vi "DEMPViewer.vi"() -> ()   [LabVIEW 2024]
uses:
  <vilib>/Utility/file.llb/Write Delimited Spreadsheet (string).vi
  E:/CodeProjects/DEMPViewer/ClassLibrary1.dll
  ClassLibrary1.dll
panel:
  out "SelectedAnalytes":string[](array[string])
  in  "Analytes":i32[](listbox)
  in  "Maximum":dbl=70.0
  in  "X Limits":bool
  in  "Minimum":dbl
  in  "Copy":bool
  out "Table Control":string[][](table)
  out "Y Scale":i64
  out "Selected Bias":i64
  in  "Clip Ends":bool=TRUE
  in  "10 nA":bool
  in  "5nA":bool
  in  "3nA":bool
  in  "1nA":bool
  in  "Y Limits":bool
  in  "500 mV":bool
  in  "100 mV":bool
  in  "50 mV":bool
  in  "10 mV":bool
  in  "Bias":bool
  in  "SaveDown":bool
  in  "LoadDown":bool
  out "Currently Loading":string
  in  "Refresh":bool
  out "Bias Graph":cluster{dbl[], "Data":dbl[]}[](graph)
  out "XY Graph 32":cluster{dbl[], "Data":dbl[]}[](graph)
  out "XY Graph 31":cluster{dbl[], "Data":dbl[]}[](graph)
  out "XY Graph 30":cluster{dbl[], "Data":dbl[]}[](graph)
  out "XY Graph 29":cluster{dbl[], "Data":dbl[]}[](graph)
  out "XY Graph 28":cluster{dbl[], "Data":dbl[]}[](graph)
  out "XY Graph 27":cluster{dbl[], "Data":dbl[]}[](graph)
  out "XY Graph 26":cluster{dbl[], "Data":dbl[]}[](graph)
  out "XY Graph 25":cluster{dbl[], "Data":dbl[]}[](graph)
  out "XY Graph 24":cluster{dbl[], "Data":dbl[]}[](graph)
  out "XY Graph 23":cluster{dbl[], "Data":dbl[]}[](graph)
  out "XY Graph 22":cluster{dbl[], "Data":dbl[]}[](graph)
  out "XY Graph 21":cluster{dbl[], "Data":dbl[]}[](graph)
  out "XY Graph 20":cluster{dbl[], "Data":dbl[]}[](graph)
  out "XY Graph 19":cluster{dbl[], "Data":dbl[]}[](graph)
  out "XY Graph 18":cluster{dbl[], "Data":dbl[]}[](graph)
  out "XY Graph 17":cluster{dbl[], "Data":dbl[]}[](graph)
  out "XY Graph 16":cluster{dbl[], "Data":dbl[]}[](graph)
  out "XY Graph 15":cluster{dbl[], "Data":dbl[]}[](graph)
  out "XY Graph 14":cluster{dbl[], "Data":dbl[]}[](graph)
  out "XY Graph 13":cluster{dbl[], "Data":dbl[]}[](graph)
  out "XY Graph 12":cluster{dbl[], "Data":dbl[]}[](graph)
  out "XY Graph 11":cluster{dbl[], "Data":dbl[]}[](graph)
  out "XY Graph 10":cluster{dbl[], "Data":dbl[]}[](graph)
  out "XY Graph 9":cluster{dbl[], "Data":dbl[]}[](graph)
  out "XY Graph 3":cluster{dbl[], "Data":dbl[]}[](graph)
  out "XY Graph 8":cluster{dbl[], "Data":dbl[]}[](graph)
  out "XY Graph 7":cluster{dbl[], "Data":dbl[]}[](graph)
  out "XY Graph 6":cluster{dbl[], "Data":dbl[]}[](graph)
  out "XY Graph 5":cluster{dbl[], "Data":dbl[]}[](graph)
  out "XY Graph 4":cluster{dbl[], "Data":dbl[]}[](graph)
  out "XY Graph 2":cluster{dbl[], "Data":dbl[]}[](graph)
  out "XY Graph 1":cluster{dbl[], "Data":dbl[]}[](graph)
  out "Loaded Files":string[](array[string])
  in  "Downsample":i32=500
  out "DataPile":T1(array[cluster])
  out "Channels":string[](array[string])
  out "Analytes":string[](array[string])
  out "dt":dbl
  in  "stop":bool
  in  "Show Conductance":bool
  in  "DEMP Folder":path
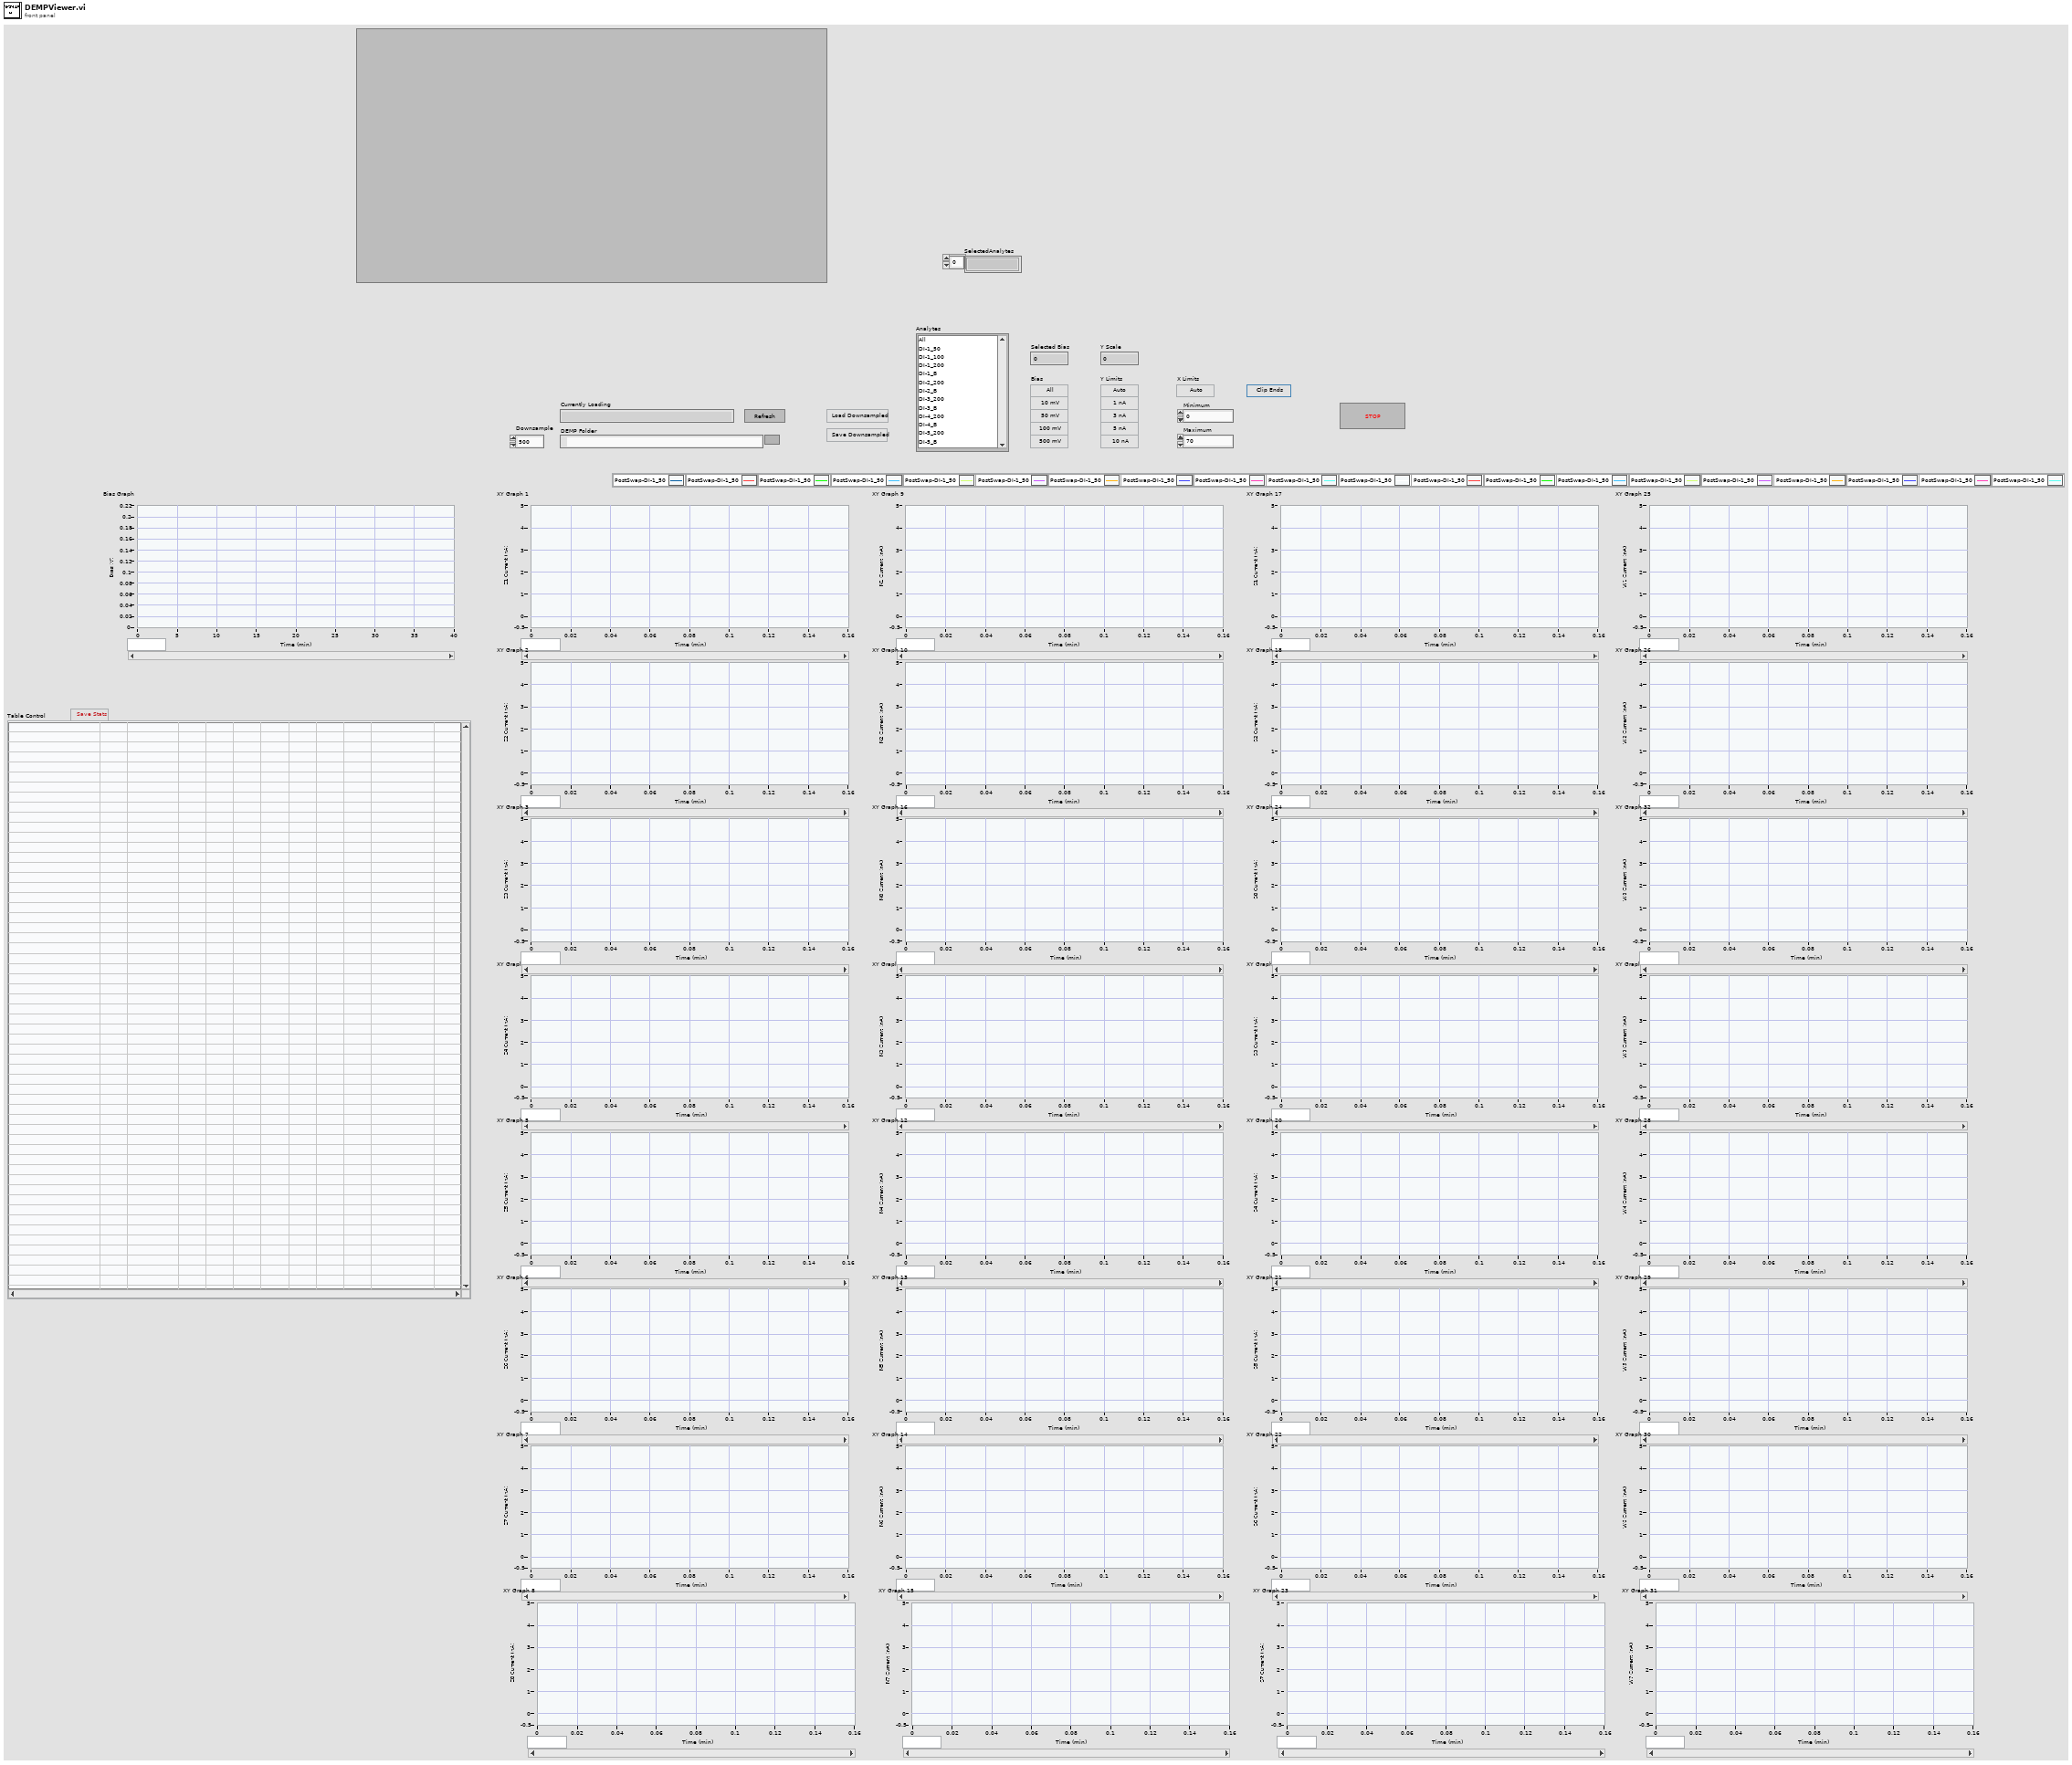
[diagram p1: front panel]
types:
  T1 = cluster{"Analyte":string, "Channel":string, "Data":dbl[], "dt":dbl}[]
  T2 = cluster{"Analyte":string, "Channel":string, "Data":dbl[], "dt":dbl}
  T3 = enum16{"open", "open or create", "create or replace", "create", "open (read-only)"}
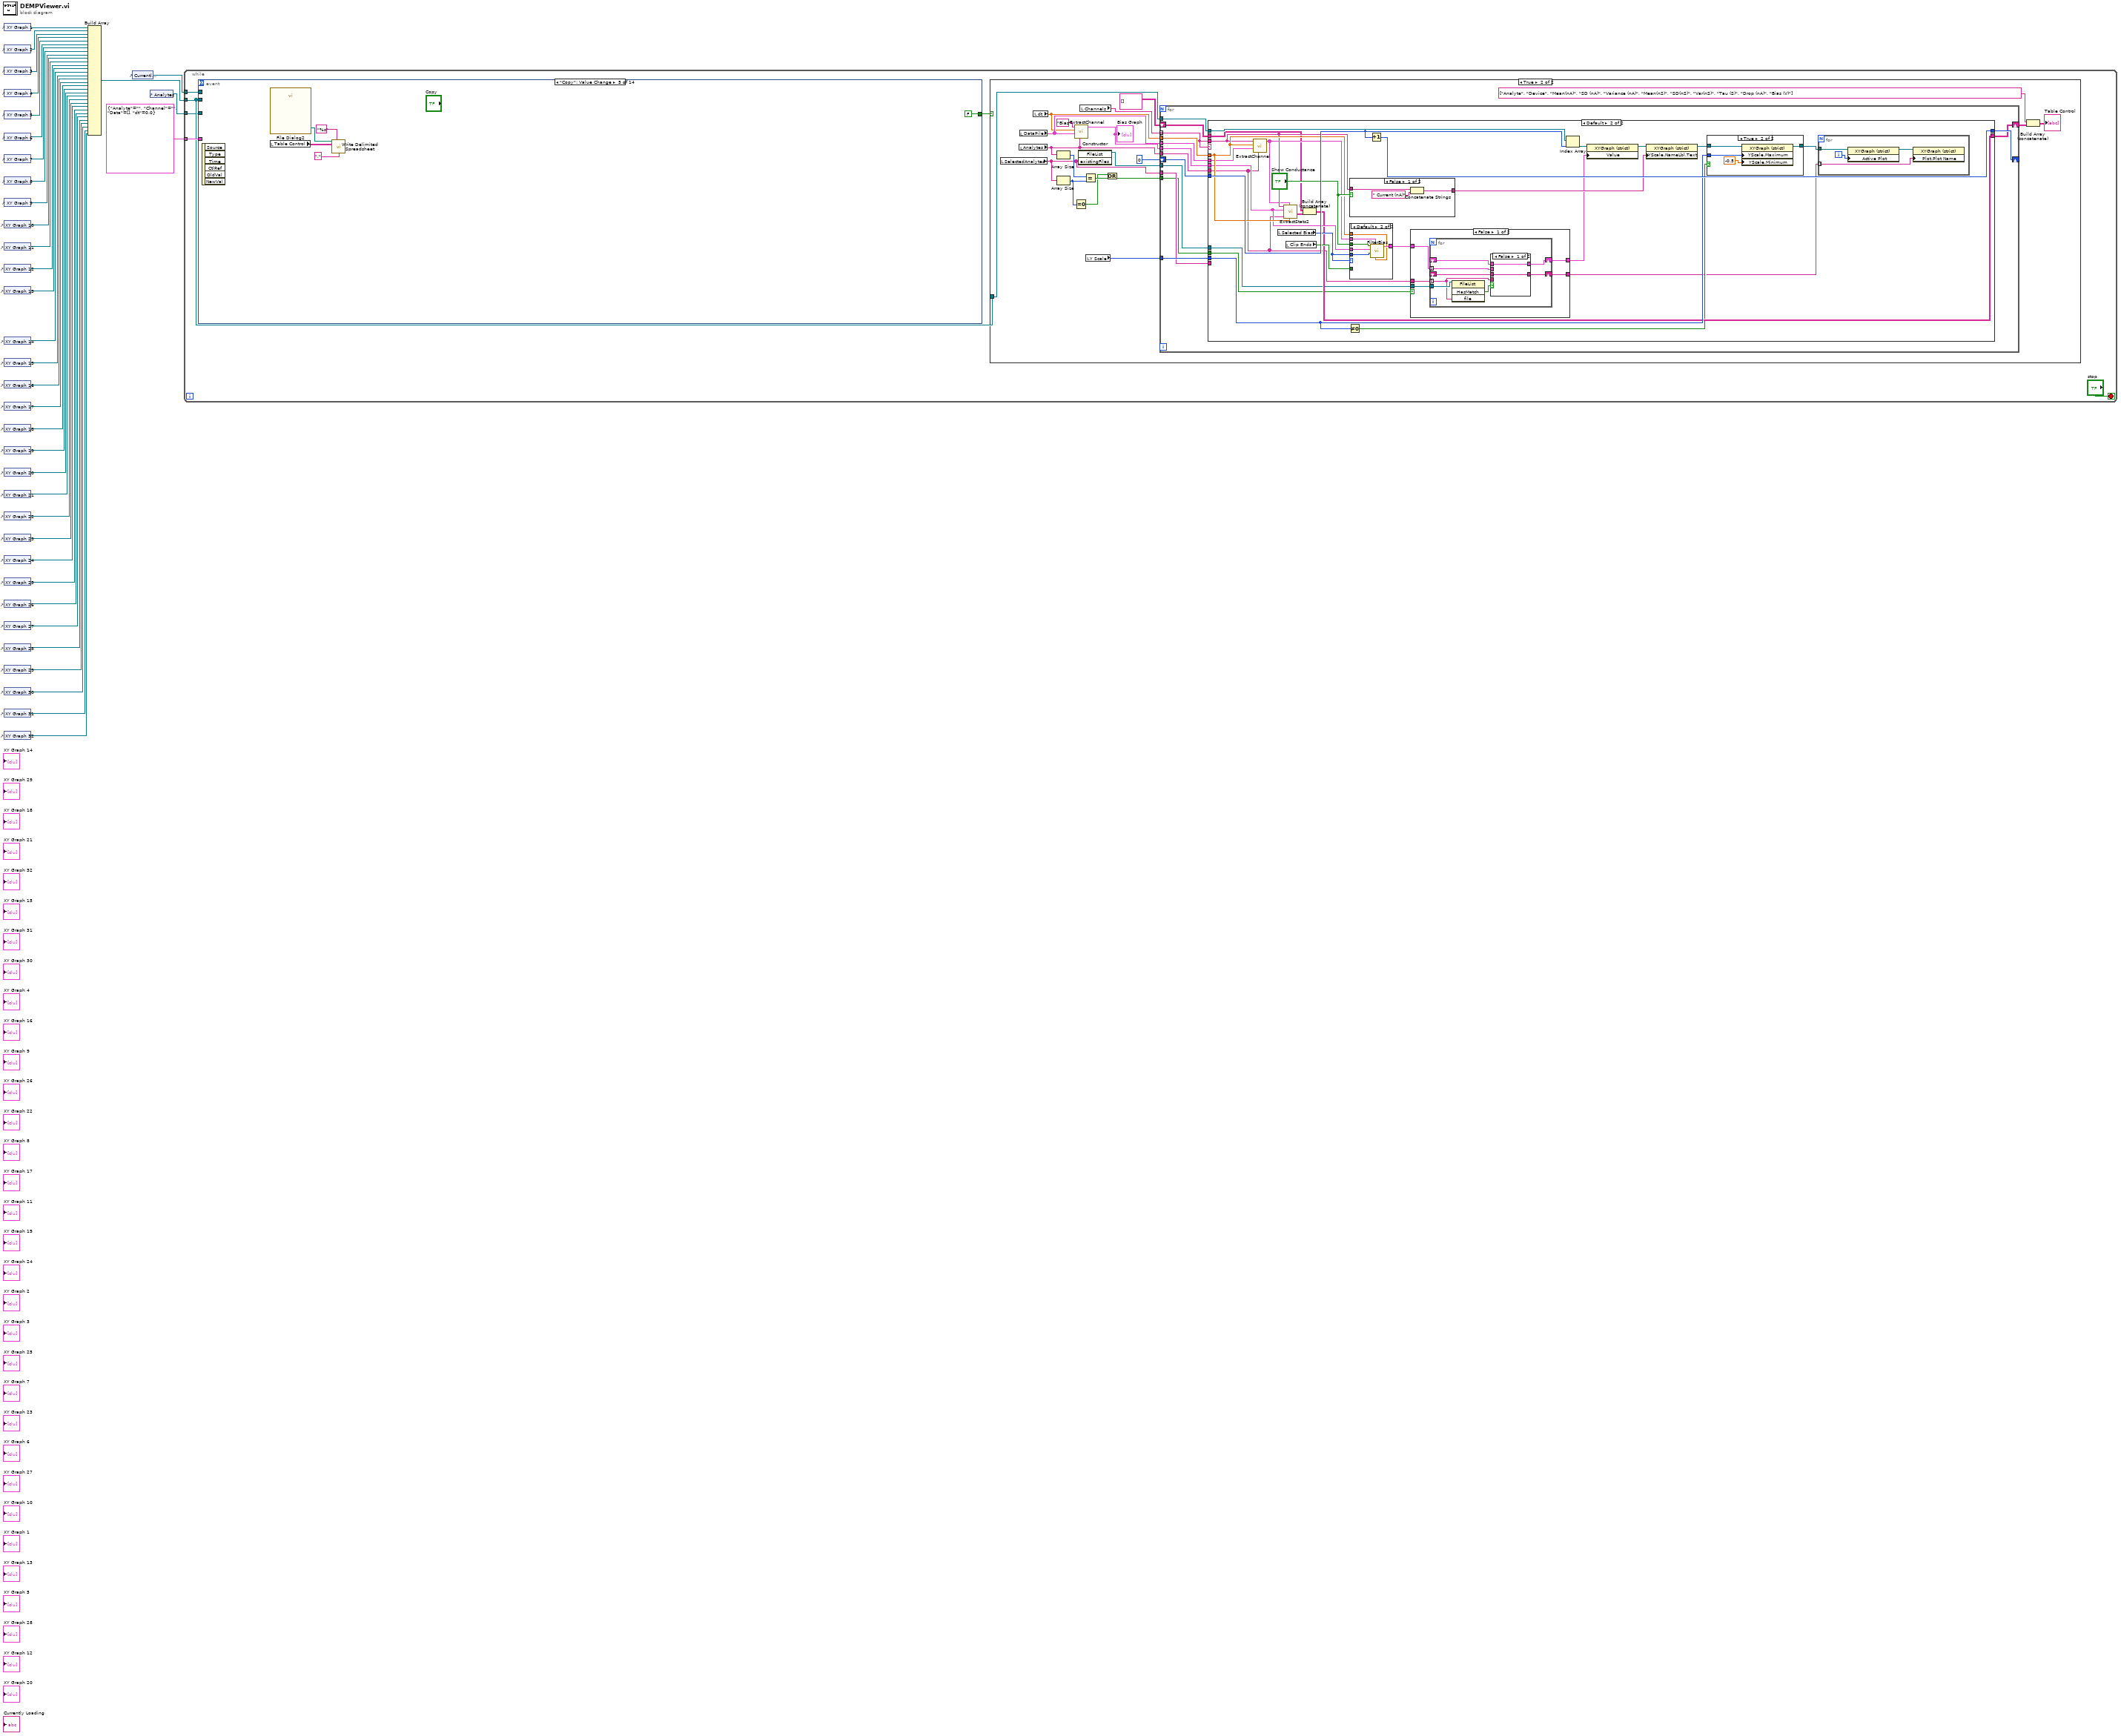
[diagram p0: block diagram]
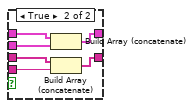
[diagram p4: hidden frame]
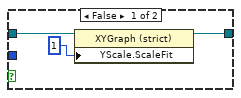
[diagram p6: hidden frame]
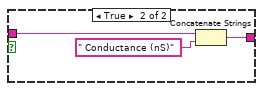
[diagram p8: hidden frame]
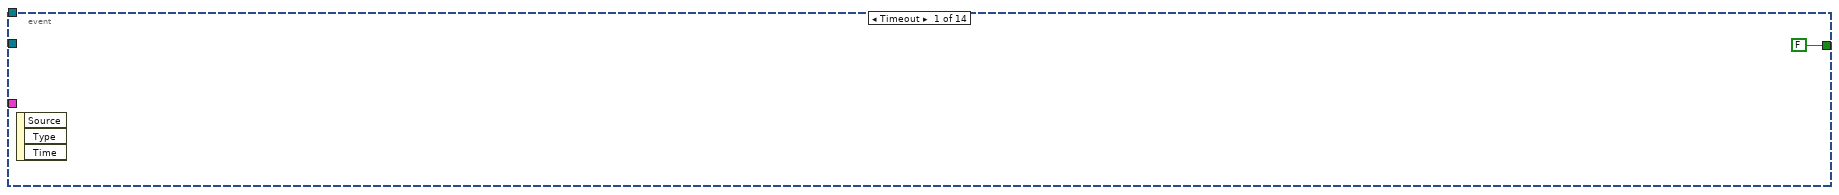
[diagram p9: hidden frame]
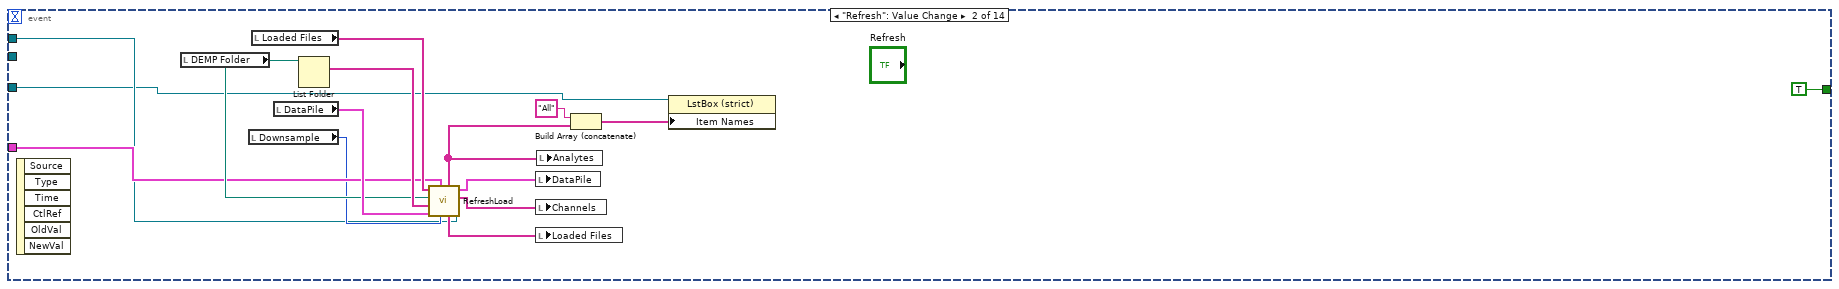
[diagram p10: hidden frame]
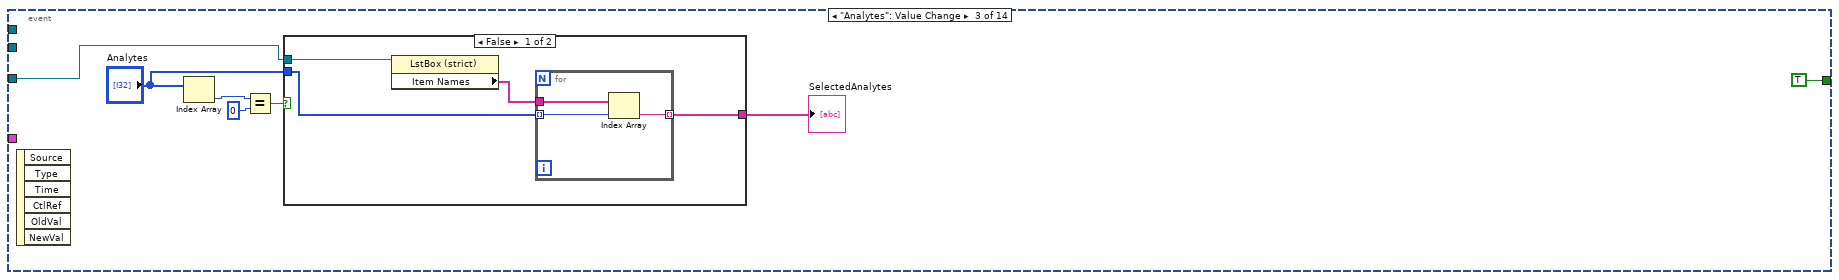
[diagram p11: hidden frame]
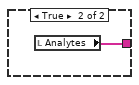
[diagram p12: hidden frame]
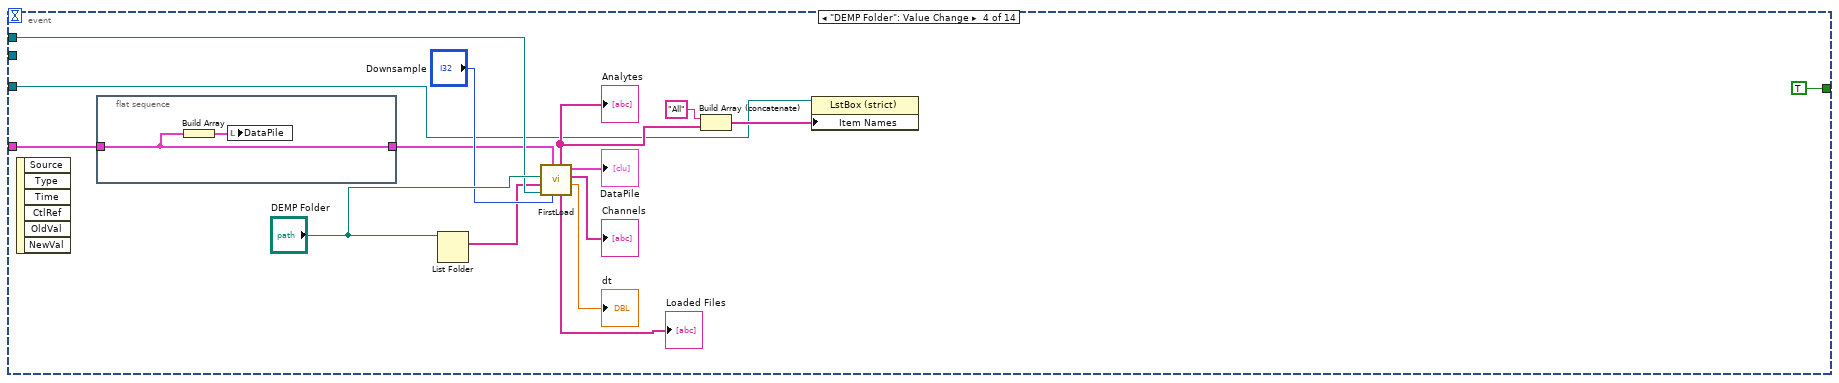
[diagram p13: hidden frame]
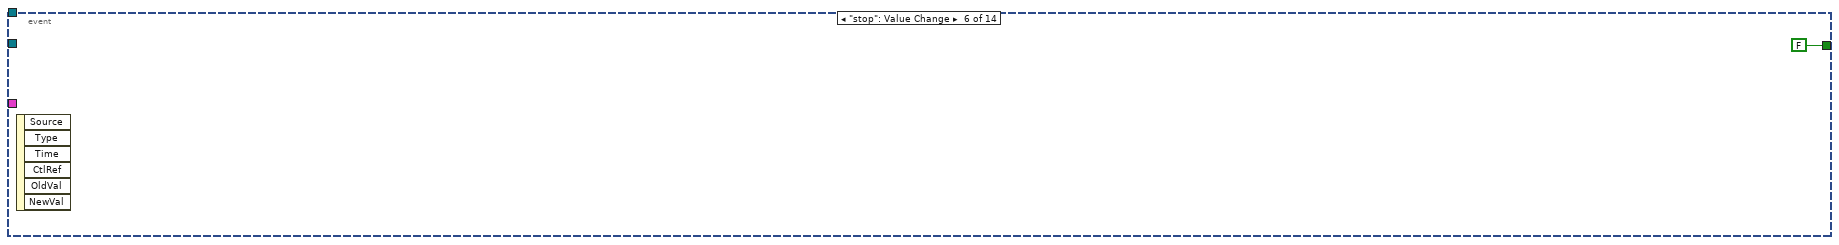
[diagram p14: hidden frame]
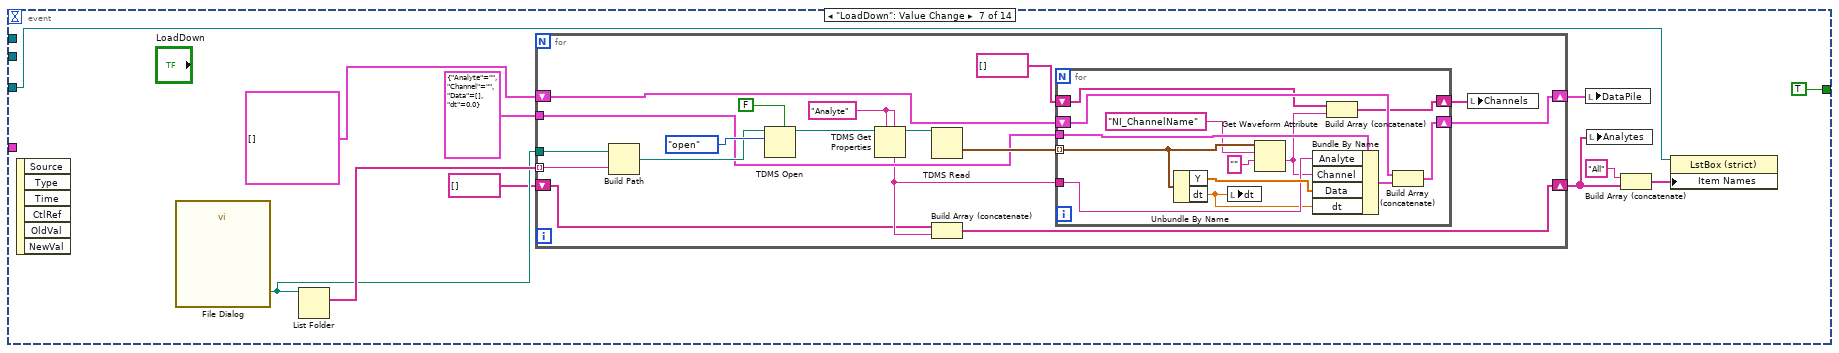
[diagram p15: hidden frame]
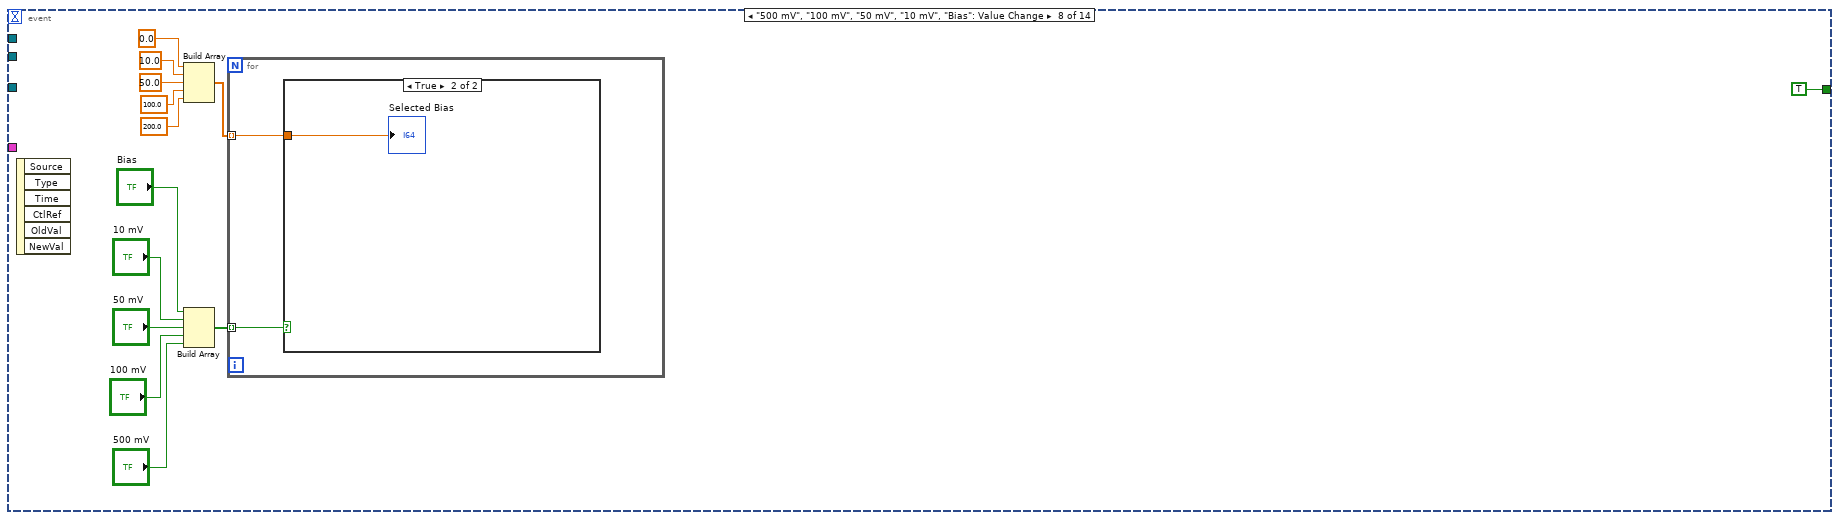
[diagram p16: hidden frame]
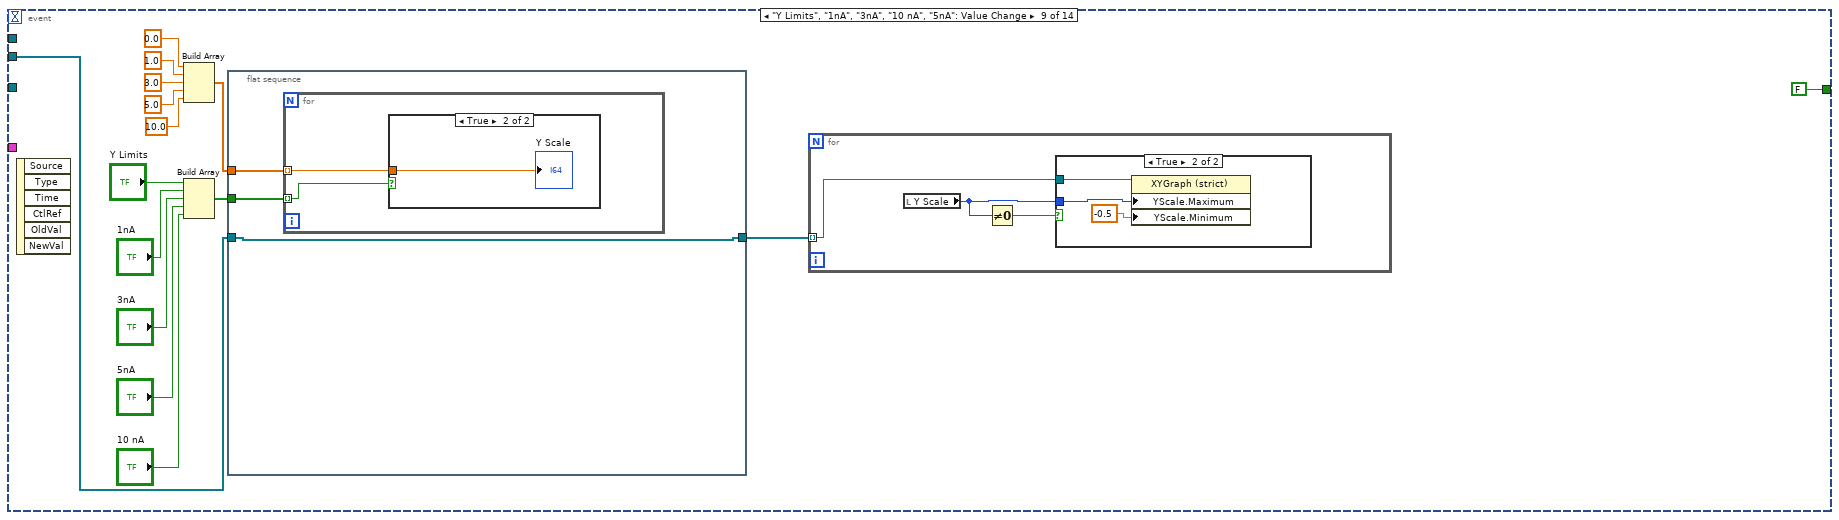
[diagram p18: hidden frame]
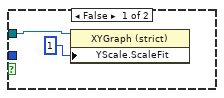
[diagram p20: hidden frame]
diagram:
  n1 = control-ref of="XY Graph 1"() -> (w35:refnum<vi>)
  n2 = control-ref of="XY Graph 2"() -> (w34:refnum<vi>)
  n3 = control-ref of="XY Graph 3"() -> (w33:refnum<vi>)
  n4 = control-ref of="XY Graph 4"() -> (w32:refnum<vi>)
  n5 = control-ref of="XY Graph 5"() -> (w31:refnum<vi>)
  n6 = control-ref of="XY Graph 6"() -> (w30:refnum<vi>)
  n7 = control-ref of="XY Graph 7"() -> (w29:refnum<vi>)
  n8 = control-ref of="XY Graph 8"() -> (w28:refnum<vi>)
  n9 = control-ref of="XY Graph 9"() -> (w27:refnum<vi>)
  n10 = control-ref of="XY Graph 10"() -> (w26:refnum<vi>)
  n11 = control-ref of="XY Graph 11"() -> (w25:refnum<vi>)
  n12 = control-ref of="XY Graph 12"() -> (w24:refnum<vi>)
  n13 = control-ref of="XY Graph 13"() -> (w23:refnum<vi>)
  n14 = control-ref of="XY Graph 14"() -> (w22:refnum<vi>)
  n15 = control-ref of="XY Graph 15"() -> (w21:refnum<vi>)
  n16 = control-ref of="XY Graph 16"() -> (w20:refnum<vi>)
  n17 = control-ref of="XY Graph 17"() -> (w19:refnum<vi>)
  n18 = control-ref of="XY Graph 18"() -> (w18:refnum<vi>)
  n19 = control-ref of="XY Graph 19"() -> (w17:refnum<vi>)
  n20 = control-ref of="XY Graph 20"() -> (w16:refnum<vi>)
  n21 = control-ref of="XY Graph 21"() -> (w15:refnum<vi>)
  n22 = control-ref of="XY Graph 22"() -> (w14:refnum<vi>)
  n23 = control-ref of="XY Graph 23"() -> (w13:refnum<vi>)
  n24 = control-ref of="XY Graph 24"() -> (w12:refnum<vi>)
  n25 = control-ref of="XY Graph 25"() -> (w11:refnum<vi>)
  n26 = control-ref of="XY Graph 26"() -> (w10:refnum<vi>)
  n27 = control-ref of="XY Graph 27"() -> (w9:refnum<vi>)
  n28 = control-ref of="XY Graph 28"() -> (w8:refnum<vi>)
  n29 = control-ref of="XY Graph 29"() -> (w7:refnum<vi>)
  n30 = control-ref of="XY Graph 30"() -> (w6:refnum<vi>)
  n31 = control-ref of="XY Graph 31"() -> (w5:refnum<vi>)
  n32 = control-ref of="XY Graph 32"() -> (w4:refnum<vi>)
  n33 = Build Array(w35, w34, w33, w32, w31, w30, w29, w28, w27, w26, w25, w24, w23, w22, w21, w20, w19, w18, w17, w16, w15, w14, w13, w12, w11, w10, w9, w8, w7, w6, w5, w4) -> (w2:refnum<vi>[])
  n34 = control-ref of="Currently Loading"() -> (w3:refnum<vi>)
  n35 = control-ref of="Analytes"() -> (w1:refnum<vi>)
  n36 = while {
    tunnel: T2 {"Analyte"="", "Channel"="", "Data"=[], "dt"=0.0} -> [w41]
    tunnel: w2 -> [w38]
    tunnel: w3 -> [w40]
    tunnel: w1 -> [w37]
    stop <- "stop" stop-if-true
    n37 = event shown="[4] \"Copy\": Value Change" {
      selector: _ -> [_ _ _ _ _ _ _ _ _ _ _ _ _ _]
      dyn-events: _ -> [_ _ _ _ _ _ _ _ _ _ _ _ _ _]
      timeout: _ -> [_ _ _ _ _ _ _ _ _ _ _ _ _ _]
      tunnel: w41 -> [_ w164 _ w190 _ _ _ _ _ _ _ _ _ _]
      tunnel: w40 -> [_ w159 _ w192 _ _ _ _ _ _ _ _ _ _]
      tunnel: [FALSE TRUE TRUE TRUE FALSE FALSE TRUE TRUE FALSE FALSE FALSE TRUE FALSE TRUE] -> w39
      tunnel: w38 -> [_ _ _ _ _ _ _ _ w264 w296 w301 _ _ _]
      tunnel: w37 -> [_ w154 w175 w184 _ _ w208 _ _ _ _ _ _ _]
      event Timeout {
        n38 = event-data() -> ()  [unwired: 1 in, 3 out]
      }
      event "Refresh": Value Change {
        n39 = event-data() -> ()  [unwired: 1 in, 6 out]
        n40 = local read "DEMP Folder"() -> (w166:path)
        n41 = local read "Downsample"() -> (w163:i32)
        n42 = local read "Loaded Files"() -> (w165:string[])
        n43 = local read "DataPile"() -> (w167:T1)
        n44 = List Folder(path=w166) -> (filenames=w168:string[])  [unwired: 3 in, 3 out]
        n45 = call "RefreshLoad.vi"("MessageBox"=w159, "Downsample"=w163, "Cluster"=w164, "DataPileIn"=w167, "FileList"=w168, "DEMP Folder"=w166, "FileListIn"=w165) -> ("Channels"=w162:string[], "DataPile"=w161:T1, "FileList"=w160:string[], "Keys"=w155:string[])  [unwired: 1 out]
        n46 = local write "DataPile"(w161) -> ()
        n47 = local write "Channels"(w162) -> ()
        n48 = local write "Loaded Files"(w160) -> ()
        n49 = local write "Analytes"(w155) -> ()
        n50 = Build Array (concatenate)("All", w155) -> (w156:string[])
        n51 = property on="Property Node" class="LstBox (strict)"(reference=w154, "Item Names"=w156) -> ()  [unwired: 1 in, 2 out]
      }
      event "Analytes": Value Change {
        n52 = event-data() -> ()  [unwired: 1 in, 6 out]
        n53 = Index Array(array="Analytes") -> (element=w173:i32)  [unwired: 1 in]
        n54 = Equal?(x=w173, y=0) -> (x = y?=w171:bool)
        n55 = case shown="False" w171 {
          tunnel: "Analytes" -> [w179 _]
          tunnel: w175 -> [w178 _]
          tunnel: [w176 w183] -> w170
          frame False {
            n56 = property on="Property Node" class="LstBox (strict)"(reference=w178) -> ("Item Names"=w177:string[])  [unwired: 1 in, 2 out]
            n57 = for {
              tunnel: w179 -> [w181] mode=indexing
              tunnel: w177 -> [w182]
              tunnel: [w180] -> w176 mode=indexing
              n58 = Index Array(array=w182, index=w181) -> (element=w180:string)
            }
          }
          frame True {
            n59 = local read "Analytes"() -> (w183:string[])
          }
        }
        "SelectedAnalytes" <- w170
      }
      event "DEMP Folder": Value Change {
        n60 = event-data() -> ()  [unwired: 1 in, 6 out]
        n61 = flat-sequence {
          tunnel: [w200] -> w189
          tunnel: w190 -> [w200]
          frame #0 {
            n62 = Build Array(w200) -> (w199:T1)
            n63 = local write "DataPile"(w199) -> ()
          }
        }
        n64 = List Folder(path="DEMP Folder") -> (filenames=w191:string[])  [unwired: 3 in, 3 out]
        n65 = call "FirstLoad.vi"("Downsample"="Downsample", "Cluster"=w189, "MessageBox"=w192, "FileList"=w191, "DEMP Folder"="DEMP Folder") -> ("dt"=→"dt":dbl, "Channels"=→"Channels":string[], "DataPile"=→"DataPile":T1, "LoadedFiles"=→"Loaded Files":string[], "Keys"=w185:string[])  [unwired: 2 in]
        "Analytes" <- w185
        n66 = Build Array (concatenate)("All", w185) -> (w186:string[])
        n67 = property on="Property Node" class="LstBox (strict)"(reference=w184, "Item Names"=w186) -> ()  [unwired: 1 in, 2 out]
      }
      event "Copy": Value Change {
        n68 = event-data() -> ()  [unwired: 1 in, 6 out]
        n69 = call "File Dialog2"() -> ("selected path"=w205:path)  [unwired: 12 in, 3 out]
        n70 = local read "Table Control"() -> (w204:string[][])
        n71 = call-poly <vilib>:"Write Delimited Spreadsheet.vi"("file path (dialog if empty)"=w205, "format (%s)"="%s", "2D data"=w204, "delimiter (\\t)"="," ("delimiter (\\t)")) -> ()  [unwired: 10 in, 2 out]
      }
      event "stop": Value Change {
        n72 = event-data() -> ()  [unwired: 1 in, 6 out]
      }
      event "LoadDown": Value Change {
        n73 = event-data() -> ()  [unwired: 1 in, 6 out]
        n74 = call "File Dialog"() -> ("selected path"=w216:path)  [unwired: 12 in, 3 out]
        n75 = List Folder(path=w216) -> (filenames=w217:string[])  [unwired: 3 in, 3 out]
        n76 = for {
          tunnel: w217 -> [w231] mode=indexing
          tunnel: w216 -> [w232]
          tunnel: T2 {"Analyte"="", "Channel"="", "Data"=[], "dt"=0.0} ("element") -> [w225]
          shift-right: [w224] -> w213
          shift-left: T1 [] -> [w223]
          shift-right: [w221] -> w210
          shift-left: string[] [] -> [w220]
          w228 = "Analyte"
          n77 = Build Path(base path=w232, name or relative path=w231) -> (appended path=w230:path)
          n78 = TDMS Open(5:FALSE ("create index file? (T)"), 10:T3."open" ("operation (0:open)"), 11:w230) -> (3:w229:refnum<k34>)  [unwired: 4 in, 1 out]
          n79 = TDMS Get Properties(5:w228, 7:w228, 11:w229) -> (3:w227:refnum<k34>, 4:w222:string)  [unwired: 3 in, 4 out]
          n80 = TDMS Read(0:w227) -> (10:w226:waveform(dbl)[])  [unwired: 7 in, 5 out]
          n81 = Build Array (concatenate)(w220, w222) -> (w221:string[])
          n82 = for {
            tunnel: w226 -> [w244] mode=indexing
            tunnel: w225 -> [w247]
            tunnel: w222 -> [w245]
            shift-right: [w240] -> w224
            shift-left: w223 -> [w239]
            shift-right: [w236] -> w218
            shift-left: string[] [] -> [w237]
            n83 = Unbundle By Name(w244) -> ("Y"=w246:dbl[], "dt"=w235:dbl)
            n84 = local write "dt"(w235) -> ()
            n85 = Get Waveform Attribute(5:"", 6:"NI_ChannelName" ("name"), 7:w244) -> (1:w238:string)  [unwired: 1 in, 3 out]
            n86 = Bundle By Name(cluster=w247, "Analyte"=w245, "Channel"=w238, "Data"=w246, "dt"=w235) -> (w241:T2)
            n87 = Build Array (concatenate)(w237, w238) -> (w236:string[])
            n88 = Build Array (concatenate)(w239, w241) -> (w240:T1)
          }
          n89 = local write "Channels"(w218) -> ()
        }
        n90 = local write "DataPile"(w213) -> ()
        n91 = local write "Analytes"(w210) -> ()
        n92 = Build Array (concatenate)("All", w210) -> (w207:string[])
        n93 = property on="Property Node" class="LstBox (strict)"(reference=w208, "Item Names"=w207) -> ()  [unwired: 1 in, 2 out]
      }
      event "500 mV", "100 mV", "50 mV", "10 mV", "Bias": Value Change {
        n94 = event-data() -> ()  [unwired: 1 in, 6 out]
        n95 = Build Array(0.0 ("element"), 10.0 ("element"), 50.0 ("element"), 100.0 ("element"), 200.0 ("element")) -> (w254:dbl[])
        n96 = Build Array("Bias", "10 mV", "50 mV", "100 mV", "500 mV") -> (w255:bool[])
        n97 = for {
          tunnel: w255 -> [w262] mode=indexing
          tunnel: w254 -> [w261] mode=indexing
          n98 = case shown="True" w262 {
            tunnel: w261 -> [_ w263]
            frame False {
            }
            frame True {
              "Selected Bias" <- w263
            }
          }
        }
      }
      event "Y Limits", "1nA", "3nA", "10 nA", "5nA": Value Change {
        n99 = event-data() -> ()  [unwired: 1 in, 6 out]
        n100 = Build Array(0.0 ("element"), 1.0 ("element"), 3.0 ("element"), 5.0 ("element"), 10.0 ("element")) -> (w277:dbl[])
        n101 = Build Array("Y Limits", "1nA", "3nA", "5nA", "10 nA") -> (w278:bool[])
        n102 = flat-sequence {
          tunnel: w278 -> [w281]
          tunnel: w277 -> [w280]
          tunnel: [w279] -> w265
          tunnel: w264 -> [w279]
          frame #0 {
            n103 = for {
              tunnel: w281 -> [w283] mode=indexing
              tunnel: w280 -> [w282] mode=indexing
              n104 = case shown="True" w283 {
                tunnel: w282 -> [_ w284]
                frame False {
                }
                frame True {
                  "Y Scale" <- w284
                }
              }
            }
          }
        }
        n105 = for {
          tunnel: w265 -> [w285] mode=indexing
          n106 = local read "Y Scale"() -> (w286:i64)
          n107 = Not Equal To 0?(x=w286) -> (x != 0?=w287:bool)
          n108 = case shown="True" w287 {
            tunnel: w285 -> [w289 w292]
            tunnel: w286 -> [_ w291]
            frame False {
              n109 = property on="Property Node" class="XYGraph (strict)"(reference=w289, "YScale.ScaleFit"=u8 1 ("Y Scale.Scale Fit")) -> ()  [unwired: 1 in, 2 out]
            }
            frame True {
              n110 = property on="Property Node" class="XYGraph (strict)"(reference=w292, "YScale.Maximum"=w291, "YScale.Minimum"=-0.5 ("X Scale.Range:Minimum")) -> ()  [unwired: 1 in, 2 out]
            }
          }
        }
      }
      event "Minimum", "Maximum": Value Change {
        n111 = event-data() -> ()  [unwired: 1 in, 6 out]
        n112 = for {
          tunnel: w296 -> [w299] mode=indexing
          tunnel: "Minimum" -> [w298]
          tunnel: "Maximum" -> [w297]
          n113 = property on="Property Node" class="XYGraph (strict)"(reference=w299, "XScale.Minimum"=w298, "XScale.Maximum"=w297) -> ()  [unwired: 1 in, 2 out]
        }
      }
      event "X Limits": Value Change {
        n114 = event-data() -> ()  [unwired: 1 in, 6 out]
        n115 = for {
          tunnel: w301 -> [w303] mode=indexing
          n116 = property on="Property Node" class="XYGraph (strict)"(reference=w303, "XScale.ScaleFit"=2) -> ()  [unwired: 1 in, 2 out]
        }
      }
      event "Clip Ends": Value Change {
        n117 = event-data() -> ()  [unwired: 1 in, 6 out]
      }
      event "SaveDown": Value Change {
        n118 = event-data() -> ()  [unwired: 1 in, 6 out]
        n119 = local read "Analytes"() -> (w307:string[])
        n120 = local read "DataPile"() -> (w306:T1)
        n121 = call "SaveDown.vi"("DataPile"=w306, "Analytes"=w307) -> ()  [unwired: 10 in]
      }
      event "Show Conductance": Value Change {
        n122 = event-data() -> ()  [unwired: 1 in, 6 out]
      }
    }
    n123 = case shown="True" w39 {
      tunnel: w38 -> [_ w58]
      frame False {
      }
      frame True {
        n124 = local read "SelectedAnalytes"() -> (w47:string[])
        n125 = local read "Analytes"() -> (w48:string[])
        n126 = local read "DataPile"() -> (w56:T1)
        n127 = local read "dt"() -> (w55:dbl)
        n128 = Array Size(array=w48) -> (size(s)=w50:i32)
        n129 = Array Size(array=w47) -> (size(s)=w44:i32)
        n130 = call "ExtractChannel.vi"("Analytes"=w48, "DataPile"=w56, "dt"=w55, "Channel"="Bias") -> ("Graphs"=w62:cluster{dbl[], dbl[]}[])  [unwired: 7 in]
        "Bias Graph" <- w62
        n131 = Equal To 0?(x=w44) -> (x = 0?=w43:bool)
        n132 = constructor class="FileList"("existingFiles"=w47) -> (reference out=w46:refnum<k24>)  [unwired: 3 in, 3 out]
        n133 = local read "Channels"() -> (w61:string[])
        n134 = Equal?(x=w50, y=w44) -> (x = y?=w49:bool)
        n135 = local read "Y Scale"() -> (w57:i64)
        n136 = Or(x=w43, y=w49) -> (x .or. y?=w45:bool)
        n137 = for {
          tunnel: w61 -> [w76] mode=indexing
          shift-right: [w74] -> _
          shift-left: 0 -> [w75]
          tunnel: w58 -> [w73]
          tunnel: w56 -> [w72]
          tunnel: w48 -> [w71]
          tunnel: w55 -> [w70]
          tunnel: w62 -> [w69]
          tunnel: w57 -> [w68]
          shift-right: [w66] -> w52
          shift-left: string[][] [] -> [w67]
          tunnel: w47 -> [w65]
          tunnel: w45 -> [w64]
          tunnel: w46 -> [w63]
          n138 = case shown="Default" w76 {
            tunnel: w76 -> [_ w96]
            tunnel: w75 -> [w78 w103]
            tunnel: [w78 w105] -> w74
            tunnel: w73 -> [_ w104]
            tunnel: w72 -> [_ w94]
            tunnel: w71 -> [_ w82]
            tunnel: w70 -> [_ w97]
            tunnel: w69 -> [_ w95]
            tunnel: w68 -> [_ w99]
            tunnel: w67 -> [w77 w91]
            tunnel: [w77 w90] -> w66
            tunnel: w65 -> [_ _]
            tunnel: w64 -> [_ w88]
            tunnel: w63 -> [_ w87]
            frame "Bias" {
            }
            frame Default {
              n139 = call "ExtractChannel.vi"("Analytes"=w82, "DataPile"=w94, "dt"=w97, "Channel"=w96) -> ("Graphs"=w93:cluster{dbl[], dbl[]}[])  [unwired: 7 in]
              n140 = local read "Selected Bias"() -> (w100:i64)
              n141 = call "ExtractStats2.vi"("dt"=w97, "Graphs"=w93, "Analytes"=w82, "Bias"=w95, "channel"=w96) -> ("dataTable"=w92:string[][])  [unwired: 6 in]
              n142 = local read "Clip Ends"() -> (w98:bool)
              n143 = Build Array (concatenate)(w91, w92) -> (w90:string[][])
              n144 = Not Equal To 0?(x=w99) -> (x != 0?=w89:bool)
              n145 = case shown="False" "Show Conductance" {
                tunnel: w96 -> [w148 w152]
                tunnel: [w147 w150] -> w102
                frame False {
                  n146 = Concatenate Strings(w148, " Current (nA)" ("string")) -> (w147:string)
                }
                frame True {
                  n147 = Concatenate Strings(w152, " Conductance (nS)" ("string")) -> (w150:string)
                }
              }
              n148 = case shown="Default" w100 {
                tunnel: [w140 w144] -> w84
                tunnel: w93 -> [w140 w145]
                tunnel: w95 -> [_ w146]
                tunnel: w97 -> [_ w143]
                tunnel: w100 -> [_ w142]
                tunnel: "Show Conductance" -> [_ w141]
                tunnel: w98 -> [_ _]
                frame 0 {
                }
                frame Default {
                  n149 = call "FilterBias.vi"("dt"=w143, "Graphs"=w145, "TargetBias"=w142, "Bias"=w146, "Show Conductance"=w141) -> ("Graphs"=w144:cluster{dbl[], dbl[]}[])  [unwired: 6 in]
                }
              }
              n150 = Increment(x=w103) -> (x+1=w105:i32)
              n151 = case shown="False" w88 {
                tunnel: w87 -> [w114 _]
                tunnel: [w111 w132] -> w85
                tunnel: w84 -> [w112 w132]
                tunnel: [w110 w131] -> w83
                tunnel: w82 -> [w113 w131]
                frame False {
                  n152 = for {
                    tunnel: w114 -> [w122]
                    tunnel: w113 -> [w118] mode=indexing
                    tunnel: w112 -> [w115] mode=indexing
                    shift-right: [w120] -> w110
                    shift-left: _ -> [w117]
                    shift-right: [w119] -> w111
                    shift-left: _ -> [w116]
                    n153 = invoke class="FileList" method="HasMatch"(reference=w122, "file"=w118) -> ("HasMatch"=w121:bool)  [unwired: 2 in, 3 out]
                    n154 = case shown="False" w121 {
                      tunnel: [w124 w130] -> w120
                      tunnel: [w123 w129] -> w119
                      tunnel: w118 -> [_ w128]
                      tunnel: w117 -> [w124 w127]
                      tunnel: w116 -> [w123 w126]
                      tunnel: w115 -> [_ w125]
                      frame False {
                      }
                      frame True {
                        n155 = Build Array (concatenate)(w126, w125) -> (w129:cluster{dbl[], dbl[]}[])
                        n156 = Build Array (concatenate)(w127, w128) -> (w130:string[])
                      }
                    }
                  }
                }
                frame True {
                }
              }
              n157 = Index Array(array=w104, index=w103) -> (element=w86:refnum<vi>)
              n158 = property on="Property Node" class="XYGraph (strict)"(reference=w86, "Value"=w85) -> (reference out=w81:refnum<vi>)  [unwired: 1 in, 1 out]
              n159 = property on="Property Node" class="XYGraph (strict)"(reference=w81, "YScale.NameLbl.Text"=w102) -> (reference out=w80:refnum<vi>)  [unwired: 1 in, 1 out]
              n160 = case shown="True" w89 {
                tunnel: w80 -> [w135 w139]
                tunnel: w99 -> [_ w138]
                tunnel: [w133 w136] -> w79
                frame False {
                  n161 = property on="Property Node" class="XYGraph (strict)"(reference=w135, "YScale.ScaleFit"=u8 1 ("Y Scale.Scale Fit")) -> (reference out=w133:refnum<vi>)  [unwired: 1 in, 1 out]
                }
                frame True {
                  n162 = property on="Property Node" class="XYGraph (strict)"(reference=w139, "YScale.Maximum"=w138, "YScale.Minimum"=-0.5 ("X Scale.Range:Minimum")) -> (reference out=w136:refnum<vi>)  [unwired: 1 in, 1 out]
                }
              }
              n163 = for {
                tunnel: w79 -> [w109]
                tunnel: w83 -> [w106] mode=indexing
                i -> [w107]
                n164 = property on="Property Node" class="XYGraph (strict)"(reference=w109, "Active Plot"=w107) -> (reference out=w108:refnum<vi>)  [unwired: 1 in, 1 out]
                n165 = property on="Property Node" class="XYGraph (strict)"(reference=w108, "Plot.Plot Name"=w106) -> ()  [unwired: 1 in, 2 out]
              }
            }
          }
        }
        n166 = Build Array (concatenate)(string[] ["Analyte", "Device", "Mean(nA)", "SD (nA)", "Variance (nA)", "Mean(nS)", "SD(nS)", "Var(nS)", "Tau (S)", "Drop (nA)", "Bias (V)"], w52) -> (→"Table Control":string[][])
      }
    }
  }
